vi "XMLStatusMessage.vi"(8 "error in (no error)":errorcluster caption="错误输入（无错误）", 9 "数组":string[](array[string]), 10 "StatusCode":string="FAIL", 11 "SerialNumber":string) -> (0 "error out":errorcluster caption="错误输出", 3 "连接的字符串":string)   [LabVIEW 2018]
uses:
  Subvi/Global.vi
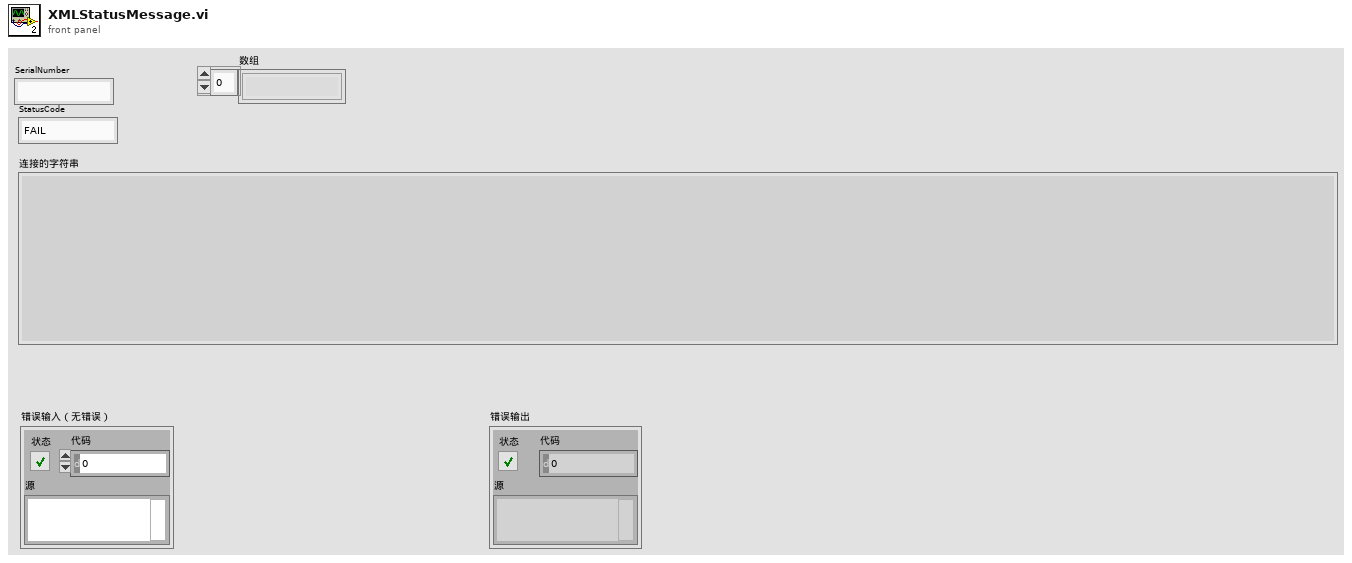
[diagram p1: front panel]
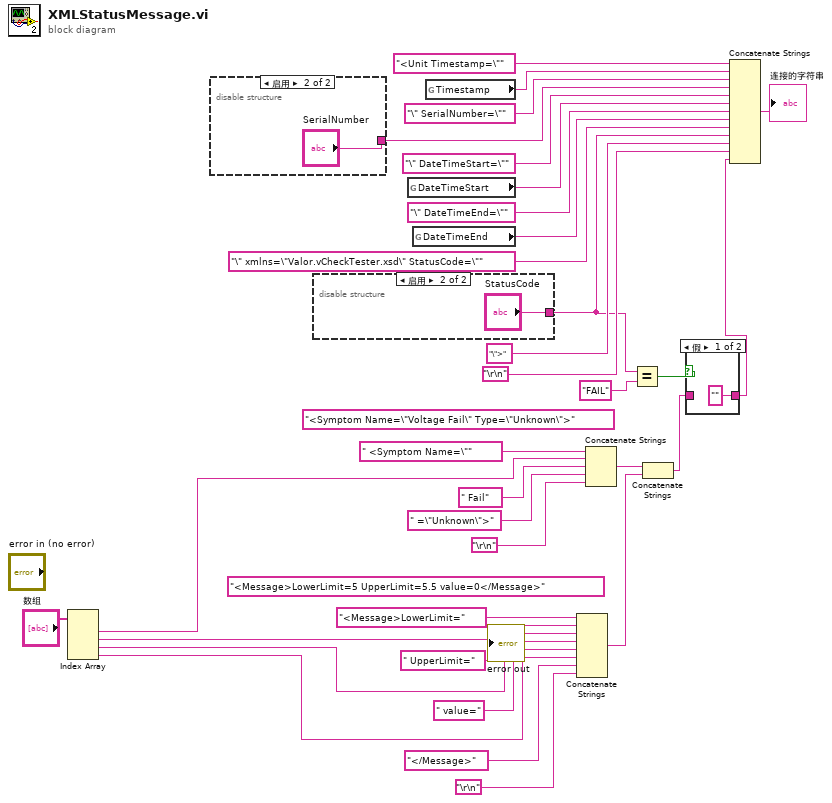
[diagram p0: block diagram]
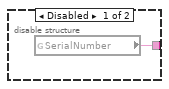
[diagram p3: hidden frame]
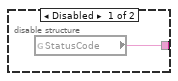
[diagram p4: hidden frame]
diagram:
  (unwired) "<Message>LowerLimit=5 UpperLimit=5.5 value=0</Message>"
  (unwired) "<Symptom Name=\"Voltage Fail\" Type=\"Unknown\">"
  n1 = Index Array(array="数组") -> (element #1=w1:string, element #2=w4:string, element #3=w3:string, element #4=w2:string)  [unwired: 4 in]
  n2 = disable-structure shown="启用" {
    disable-tunnel: [w34 "SerialNumber"] -> w30
    frame Disabled {
      n3 = global read "Global.vi" "SerialNumber"() -> (w34:string)
    }
    frame Enabled {
    }
  }
  n4 = disable-structure shown="启用" {
    disable-tunnel: [w36 "StatusCode"] -> w11
    frame Disabled {
      n5 = global read "Global.vi" "StatusCode"() -> (w36:string)
    }
    frame Enabled {
    }
  }
  n6 = global read "Global.vi" "DateTimeStart"() -> (w28:string)
  n7 = global read "Global.vi" "DateTimeEnd"() -> (w26:string)
  n8 = global read "Global.vi" "Timestamp"() -> (w32:string)
  n9 = Concatenate Strings("<Message>LowerLimit=", w4, " UpperLimit=", w3, " value=", w2, "</Message>", "\r\n") -> (w9:string)
  n10 = Concatenate Strings(" <Symptom Name=\"", w1, " Fail", " =\"Unknown\">", "\r\n") -> (w10:string)
  n11 = Equal?(x=w11, y="FAIL") -> (x = y?=w7:bool)
  n12 = Concatenate Strings(w10, w9) -> (w8:string)
  n13 = case shown="假" w7 {
    tunnel: w8 -> [_ w39]
    tunnel: ["" w39] -> w6
    frame False {
    }
    frame True {
    }
  }
  n14 = Concatenate Strings("<Unit Timestamp=\"", w32, "\" SerialNumber=\"", w30, "\" DateTimeStart=\"", w28, "\" DateTimeEnd=\"", w26, "\" xmlns=\"Valor.vCheckTester.xsd\" StatusCode=\"", w11, "\">", "\r\n", w6) -> (→"连接的字符串":string)
